vi "Main.vi"() -> ()   [LabVIEW 2017, in "Application.lvlib"]
doc: "This VI is the main application VI in the Delacor QMH project template. This application VI is implemented as a simple state machine, which communicates with two different Delacor QMH modules.\n_____\nBased on Delacor QMH Project Template 3.1.0.34."
uses:
  Application.lvlib
  Application Data--cluster.ctl
  State--enum.ctl
  My Cloneable Module/My Cloneable Module.lvlib
  My Singleton Module/My Singleton Module.lvlib
panel:
  out "version":string
  in  "Hide My Singleton Module":bool
  in  "Show My Singleton Module":bool
  in  "Hide My Cloneable Module":bool
  in  "Show My Cloneable Module":bool
  in  "Stop My Cloneable Module":bool
  in  "Stop My Singleton Module":bool
  in  "Start My Singleton Module":bool
  out "Active Cloneable Modules":string[](array[string])
  in  "Start New Instance My Cloneable Module":bool
  in  "Select Cloneable Module Instance":i32(ring)=-1 items=["All"=-1]
  in  "My Singleton Module: Do Something Else":dbl caption="Do Something Else"
  in  "My Singleton Module: Do Something":bool
  out "My Singleton Running?":bool
  out "Status":string
  in  "My Cloneable Module: Do Something Else":dbl caption="Do Something Else to Selected Module"
  in  "My Cloneable Module: Do Something":bool caption="Do Something to Selected Module"
  # "This top-level application allows you to launch and control a singleton module, and multiple instances of a cloneable module."
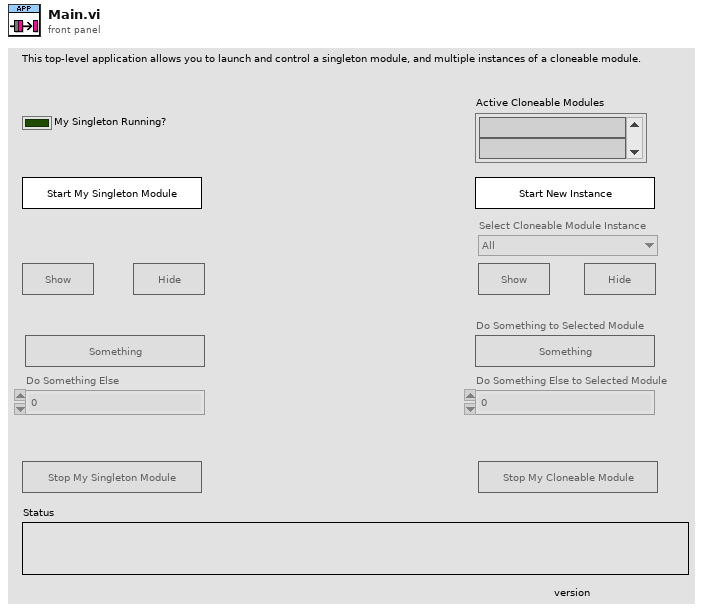
[diagram p1: front panel]
types:
  T1 = typedef "Application.lvlib/State--enum.ctl" = enum16{"Initialize", "Initialize Panel", "UI Interlocks", "Update Status", "Wait for Event", "Exit"}
  T2 = typedef "Application.lvlib/Application Data--cluster.ctl" = cluster{"Status":string, "Singleton Controls":refnum<vi>[], "Cloneable Controls":refnum<vi>[], "Module Ring Value":i32}
  T3 = typedef "My Cloneable Module.lvlib/Broadcast Events--cluster.ctl" = cluster{"Module Did Init":refnum<user-event>, "Status Updated":refnum<user-event>, "Error Reported":refnum<user-event>, "Did Something":refnum<user-event>, "Module Did Stop":refnum<user-event>, "Update Module Execution Status":refnum<user-event>}
  T4 = typedef "My Singleton Module.lvlib/Broadcast Events--cluster.ctl" = cluster{"Module Did Init":refnum<user-event>, "Status Updated":refnum<user-event>, "Error Reported":refnum<user-event>, "Did Something":refnum<user-event>, "Module Did Stop":refnum<user-event>, "Update Module Execution Status":refnum<user-event>}
  T5 = enum8{"Enabled", "Disabled", "Disabled and Grayed Out"}
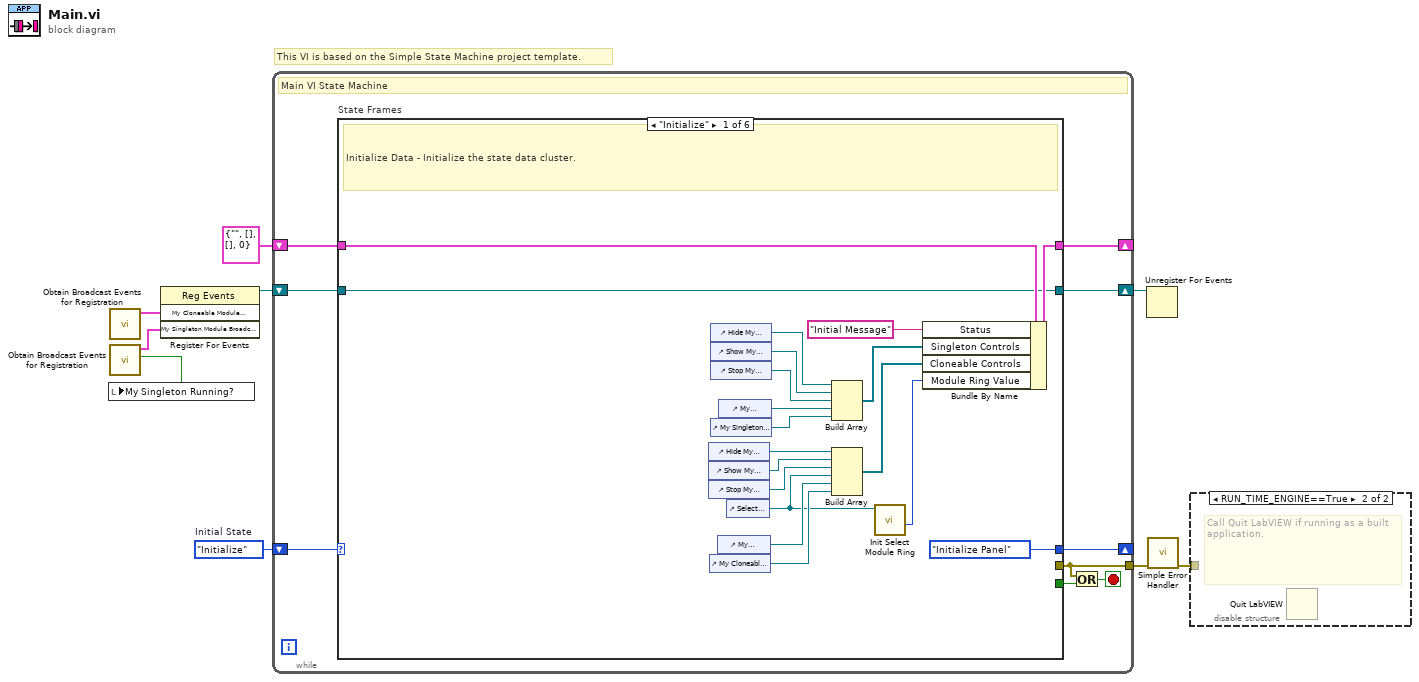
[diagram p0: block diagram]
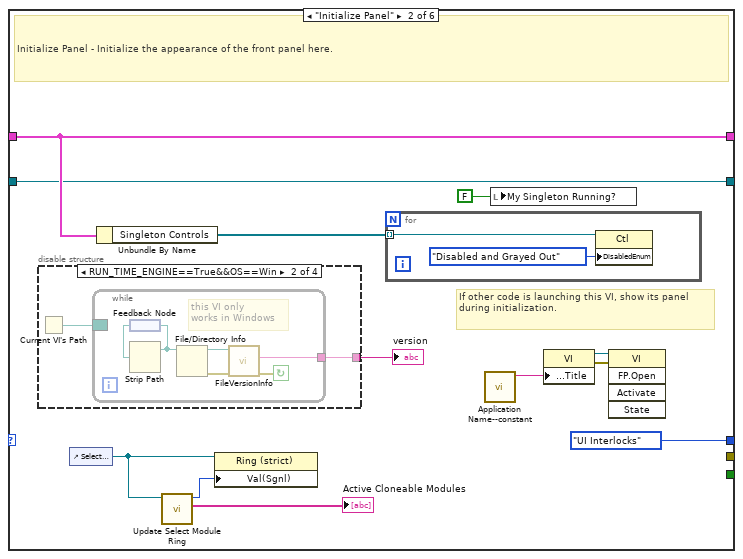
[diagram p2: hidden frame]
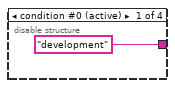
[diagram p3: hidden frame]
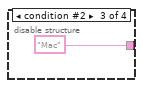
[diagram p4: hidden frame]
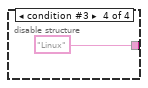
[diagram p5: hidden frame]
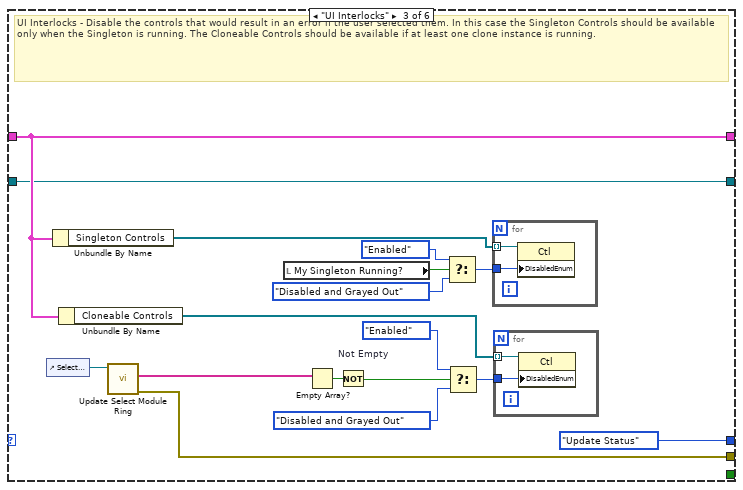
[diagram p6: hidden frame]
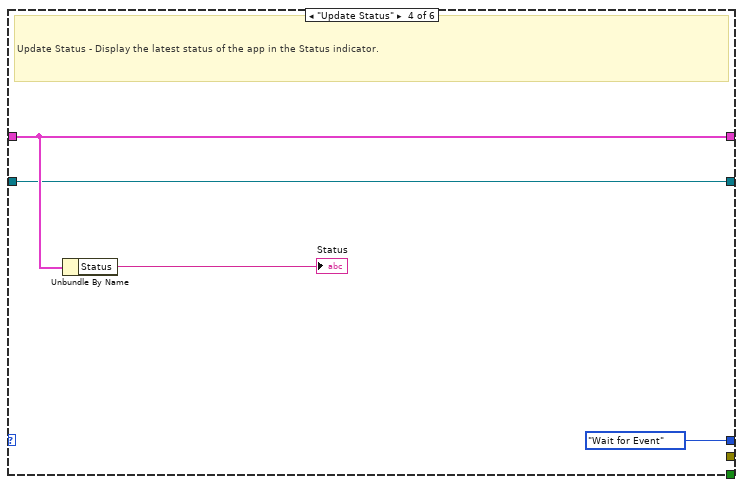
[diagram p7: hidden frame]
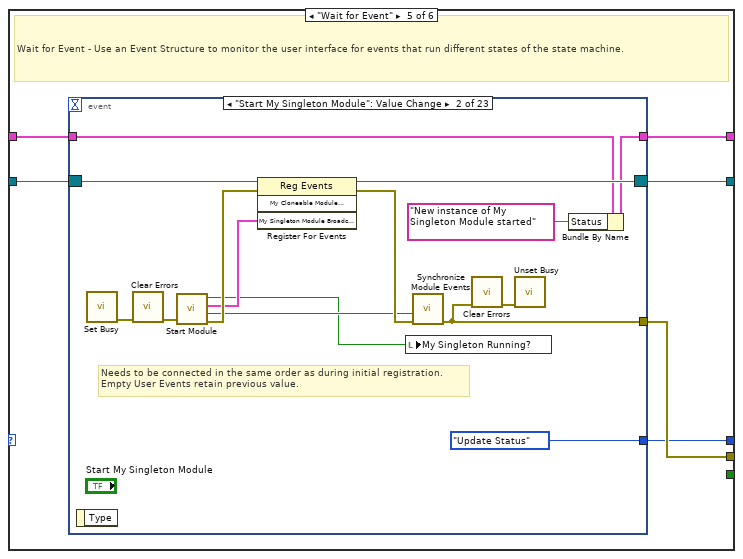
[diagram p8: hidden frame]
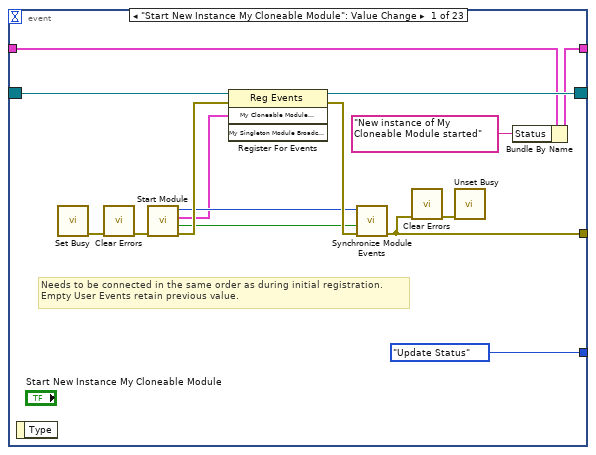
[diagram p9: hidden frame]
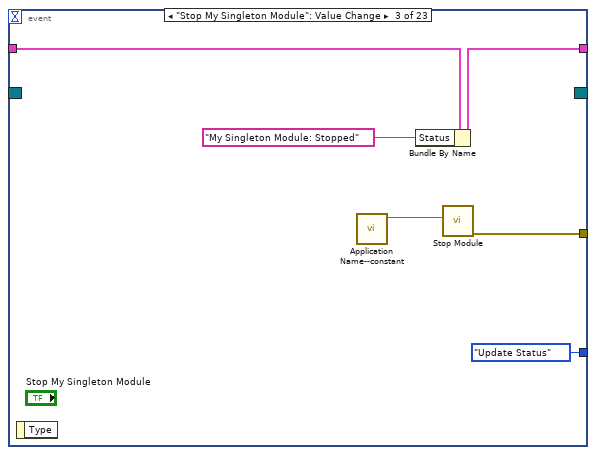
[diagram p10: hidden frame]
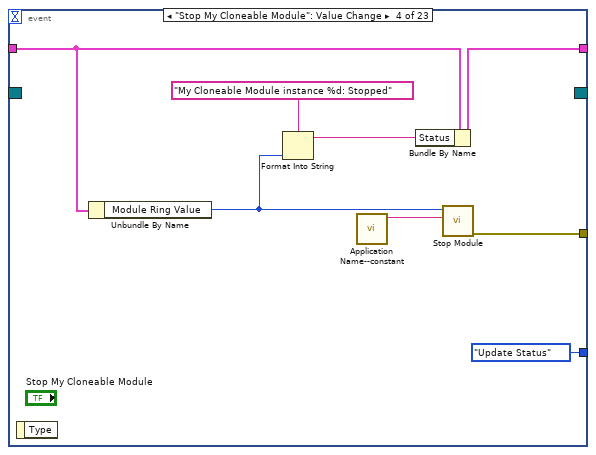
[diagram p11: hidden frame]
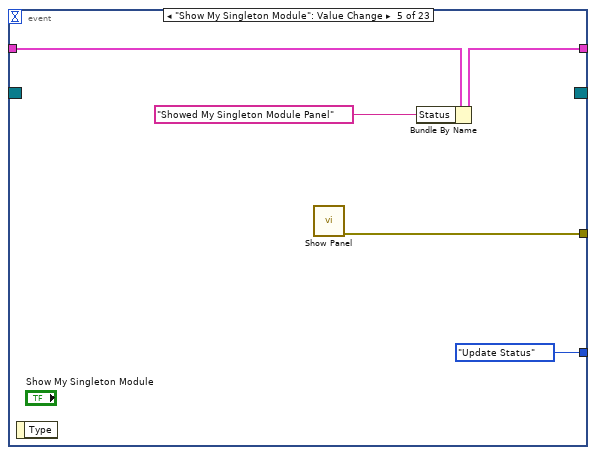
[diagram p12: hidden frame]
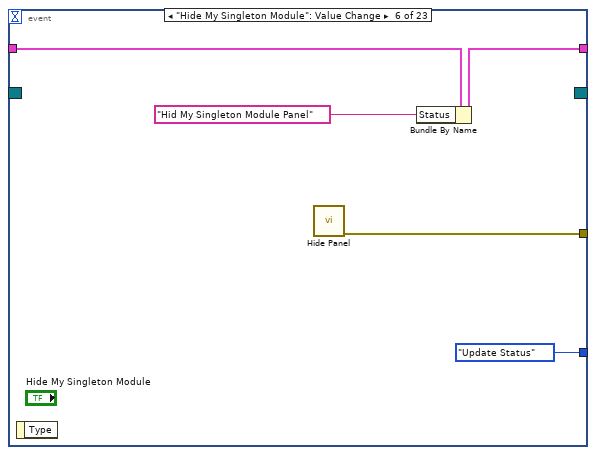
[diagram p13: hidden frame]
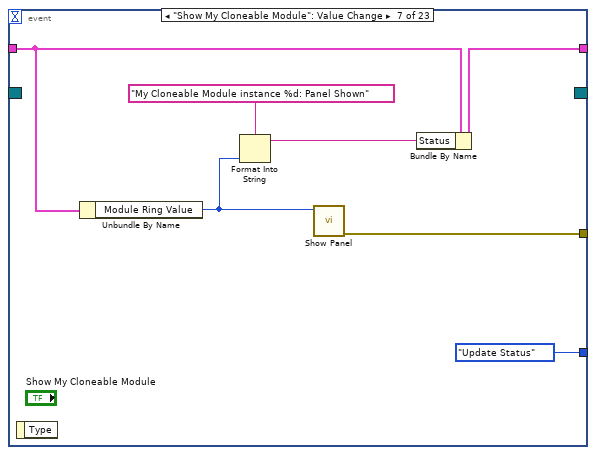
[diagram p14: hidden frame]
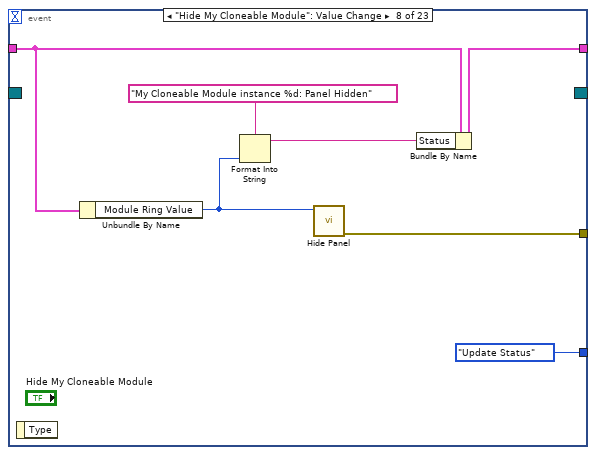
[diagram p15: hidden frame]
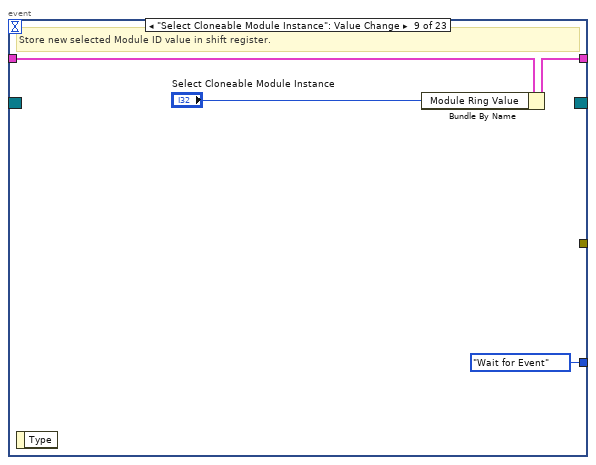
[diagram p16: hidden frame]
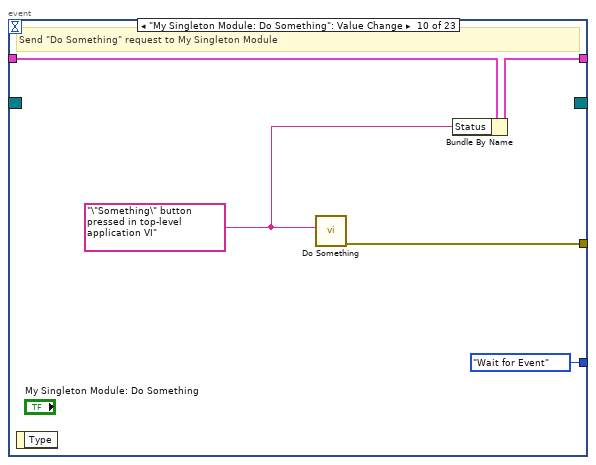
[diagram p17: hidden frame]
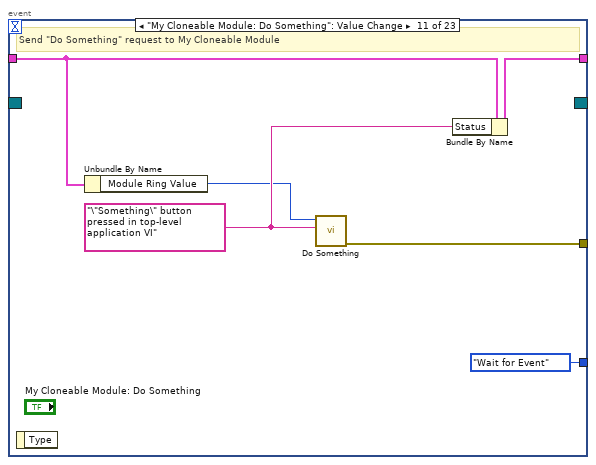
[diagram p18: hidden frame]
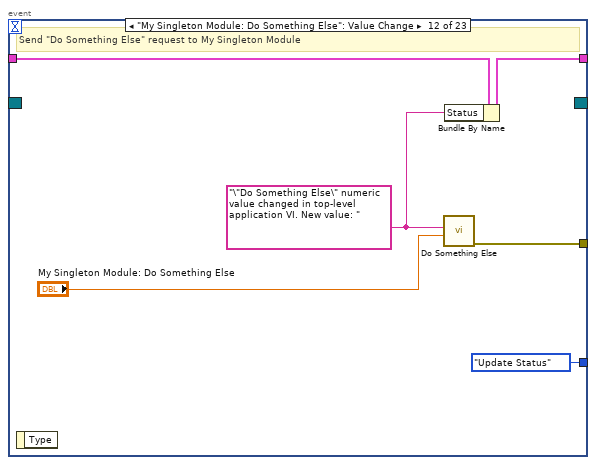
[diagram p19: hidden frame]
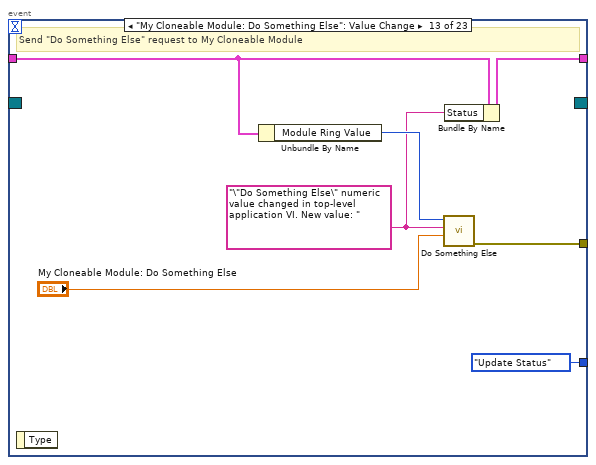
[diagram p20: hidden frame]
diagram:
  w4 = State--enum."Initialize"  # Initial State
  # "This VI is based on the Simple State Machine project template."
  n1 = call "Obtain Broadcast Events for Registration.vi"() -> ("My Cloneable Module Broadcast Events"=w8:T3)  [unwired: 10 in, 1 out]
  n2 = call "Obtain Broadcast Events for Registration.vi"() -> ("Already running?"=w1:bool, "My Singleton Module Broadcast Events"=w7:T4)  [unwired: 9 in, 1 out]
  n3 = local write "My Singleton Running?"(w1) -> ()
  n4 = register-events(w8, w7) -> (reference out=w3:refnum<event-registration>)  [unwired: 2 in, 1 out]
  n5 = while {
    shift-right: [w17] -> _
    shift-left: T2 {"Status"="", "Singleton Controls"=[], "Cloneable Controls"=[], "Module Ring Value"=0} ("Data Cluster") -> [w18]
    tunnel: [w13] -> w6
    shift-right: [w12] -> _
    shift-left: w4 -> [w15]
    shift-right: [w10] -> w2
    shift-left: w3 -> [w11]
    stop <- w14 stop-if-true
    # "Main VI State Machine"
    n6 = case "State Frames" shown="\"Initialize\"" w15 {
      tunnel: [_ _ w63 _ w89 w261] -> w13
      tunnel: w18 -> [w37 w47 w68 w87 w91 w263]
      tunnel: [w36 w47 w68 w87 w90 w263] -> w17
      tunnel: [_ _ _ _ _ w262] -> w16
      tunnel: [State--enum."Initialize Panel" ("State") State--enum."UI Interlocks" ("State") State--enum."Update Status" ("State") State--enum."Wait for Event" ("State") w88 State--enum."Exit" ("State")] -> w12
      tunnel: w11 -> [w19 w44 w64 w84 w93 w257]
      tunnel: [w19 w44 w64 w84 w92 w257] -> w10
      frame "Initialize" {
        # "Initialize Data - Initialize the state data cluster."
        n7 = control-ref of="Hide My Cloneable Module"() -> (w28:refnum<vi>)
        n8 = control-ref of="Show My Cloneable Module"() -> (w27:refnum<vi>)
        n9 = control-ref of="Stop My Cloneable Module"() -> (w26:refnum<vi>)
        n10 = control-ref of="My Cloneable Module: Do Something"() -> (w23:refnum<vi>)
        n11 = control-ref of="Hide My Singleton Module"() -> (w34:refnum<vi>)
        n12 = control-ref of="Show My Singleton Module"() -> (w33:refnum<vi>)
        n13 = control-ref of="Stop My Singleton Module"() -> (w32:refnum<vi>)
        n14 = control-ref of="My Singleton Module: Do Something"() -> (w30:refnum<vi>)
        n15 = control-ref of="My Cloneable Module: Do Something Else"() -> (w24:refnum<vi>)
        n16 = control-ref of="My Singleton Module: Do Something Else"() -> (w31:refnum<vi>)
        n17 = control-ref of="Select Cloneable Module Instance"() -> (w21:refnum<vi>)
        n18 = Build Array(w34, w33, w32, w31, w30) -> (w29:refnum<vi>[])
        n19 = Build Array(w28, w27, w26, w21, w24, w23) -> (w25:refnum<vi>[])
        n20 = call "Init Select Module Ring.vi"("Select Module Ring Ref"=w21) -> ("Module Ring Value"=w20:i32)  [unwired: 8 in, 2 out]
        n21 = Bundle By Name(cluster=w37, "Status"="Initial Message" ("Initial Message"), "Singleton Controls"=w29, "Cloneable Controls"=w25, "Module Ring Value"=w20) -> (w36:T2)
      }
      frame "Initialize Panel" {
        # "If other code is launching this VI, show its panel during initialization."
        # "Initialize Panel - Initialize the appearance of the front panel here."
        n22 = disable-structure "Conditional Disable Structure" shown="RUN_TIME_ENGINE==True&&OS==Win" {
          disable-tunnel: ["development" w51 "Mac" "Linux"] -> w41
          frame condition #0 (active) {
          }
          frame condition #1 {
            n23 = Current VI's Path() -> (path=w52:path)
            n24 = while {
              border: w52 -> [_]
              tunnel: [w53] -> w51
              stop <- w54 continue-if-true
              # "this VI only \nworks in Windows"
              n25 = feedback #1() -> (w58:path)
              n26 = Strip Path(path=w58) -> (stripped path=w57:path)  [unwired: 1 out]
              n27 = feedback-in #1(w57) -> ()
              n28 = File/Directory Info(path=w57) -> (path out=w55:path, error out=w56:errorcluster)  [unwired: 1 in, 5 out]
              n29 = call <vilib>:"FileVersionInfo.vi"("error in (no error)"=w56, "Application Path in"=w55) -> ("error out"=w54:errorcluster, "File Version Info"=w53:string)  [unwired: 6 in, 2 out]
            }
          }
          frame condition #2 {
          }
          frame condition #3 {
          }
        }
        "version" <- w41
        n30 = control-ref of="Select Cloneable Module Instance"() -> (w43:refnum<vi>)
        n31 = Unbundle By Name(w47) -> ("Singleton Controls"=w46:refnum<vi>[])
        n32 = call "Update Select Module Ring.vi"("Select Module Ring Ref"=w43) -> ("Active Modules (Array)"=→"Active Cloneable Modules":string[], "New Module Ring Value"=w42:i32)  [unwired: 8 in, 1 out]
        n33 = property on="Property Node" class="Ring (strict)"(reference=w43, "Val(Sgnl)"=w42) -> ()  [unwired: 1 in, 2 out]
        n34 = for {
          tunnel: w46 -> [w62] mode=indexing
          n35 = property on="Property Node" class="Ctl"(reference=w62, "DisabledEnum"=T5."Disabled and Grayed Out" ("Disabled")) -> ()  [unwired: 1 in, 2 out]
        }
        n36 = call "Application Name--constant.vi"() -> ("Application Name"=w40:string)  [unwired: 11 in]
        n37 = local write "My Singleton Running?"(FALSE ("My Singleton Module Init?")) -> ()
        n38 = property on="Property Node" class="VI"("Front Panel.Title"=w40) -> (reference out=w39:refnum<vi>, error out=w38:errorcluster)  [unwired: 2 in]
        n39 = invoke class="VI" method="FP.Open"(reference=w39, error in=w38) -> ()  [unwired: 3 in, 5 out]
      }
      frame "UI Interlocks" {
        # "UI Interlocks - Disable the controls that would result in an error if the user selected them. In this case the Singleton Controls should be available only when the Singleton is running. The Cloneable Controls should be available if at least one clone instance is running."
        n40 = control-ref of="Select Cloneable Module Instance"() -> (w79:refnum<vi>)
        n41 = Unbundle By Name(w68) -> ("Singleton Controls"=w73:refnum<vi>[])
        n42 = Unbundle By Name(w68) -> ("Cloneable Controls"=w67:refnum<vi>[])
        n43 = call "Update Select Module Ring.vi"("Select Module Ring Ref"=w79) -> ("error out"=w63:errorcluster, "Active Modules (Array)"=w78:string[])  [unwired: 8 in, 1 out]
        n44 = local read "My Singleton Running?"() -> (w72:bool)
        n45 = Empty Array?(array=w78) -> (empty?=w77:bool)
        n46 = Not "Not Empty"(x=w77) -> (.not. x?=w66:bool)
        n47 = Select(t=T5."Enabled" ("Disabled"), s=w72, f=T5."Disabled and Grayed Out" ("Disabled")) -> (s? t:f=w74:T5)
        n48 = Select(t=T5."Enabled" ("Disabled"), s=w66, f=T5."Disabled and Grayed Out" ("Disabled")) -> (s? t:f=w71:T5)
        n49 = for {
          tunnel: w73 -> [w83] mode=indexing
          tunnel: w74 -> [w82]
          n50 = property on="Property Node" class="Ctl"(reference=w83, "DisabledEnum"=w82) -> ()  [unwired: 1 in, 2 out]
        }
        n51 = for {
          tunnel: w67 -> [w81] mode=indexing
          tunnel: w71 -> [w80]
          n52 = property on="Property Node" class="Ctl"(reference=w81, "DisabledEnum"=w80) -> ()  [unwired: 1 in, 2 out]
        }
      }
      frame "Update Status" {
        # "Update Status - Display the latest status of the app in the Status indicator."
        n53 = Unbundle By Name(w87) -> ("Status"=→"Status":string)
      }
      frame "Wait for Event" {
        # "Wait for Event - Use an Event Structure to monitor the user interface for events that run different states of the state machine."
        n54 = event shown="[1] \"Start My Singleton Module\": Value Change" {
          selector: w93 -> [w101 w117 _ _ _ _ _ _ _ _ _ _ _ _ _ _ _ _ _ _ _ _ _]
          dyn-events: [w100 w116 _ _ _ _ _ _ _ _ _ _ _ _ _ _ _ _ _ _ _ _ _] -> w92
          timeout: _ -> [_ _ _ _ _ _ _ _ _ _ _ _ _ _ _ _ _ _ _ _ _ _ _]
          tunnel: [w108 w123 w127 w135 w142 w147 w154 w161 _ w170 w176 w182 w189 w193 w198 w204 _ _ _ _ w241 _ _] -> w89
          tunnel: [w96 w113 w125 w134 w140 w145 w153 w160 w163 w168 w175 w180 w188 w192 w200 w206 w207 w212 w223 w233 w236 w247 w252] -> w90
          tunnel: w91 -> [w97 w114 w126 w133 w141 w146 w151 w158 w164 w169 w172 w181 w186 w192 w200 w206 w208 w213 w224 w234 w239 w248 w252]
          tunnel: [State--enum."Update Status" ("State") State--enum."Update Status" ("State") State--enum."Update Status" ("State") State--enum."Update Status" ("State") State--enum."Update Status" ("State") State--enum."Update Status" ("State") State--enum."Update Status" ("State") State--enum."Update Status" ("State") State--enum."Wait for Event" ("State") State--enum."Wait for Event" ("State") State--enum."Wait for Event" ("State") State--enum."Update Status" ("State") State--enum."Update Status" ("State") State--enum."UI Interlocks" ("State") State--enum."UI Interlocks" ("State") State--enum."UI Interlocks" ("State") State--enum."Update Status" ("State") State--enum."Update Status" ("State") State--enum."Update Status" ("State") State--enum."Update Status" ("State") State--enum."UI Interlocks" ("State") State--enum."UI Interlocks" ("State") State--enum."Exit" ("State")] -> w88
          event "Start New Instance My Cloneable Module": Value Change {
            # "Needs to be connected in the same order as during initial registration.\nEmpty User Events retain previous value."
            n55 = event-data() -> ()  [unwired: 1 in, 1 out]
            n56 = call <vilib>:"Set Busy.vi"() -> ("error out"=w102:errorcluster)  [unwired: 10 in, 1 out]
            n57 = call <vilib>:"Clear Errors.vi"("error in (no error)"=w102) -> ("error out"=w103:errorcluster)  [unwired: 5 in, 1 out]
            n58 = call "Start Module.vi"("error in (no error)"=w103) -> ("error out"=w107:errorcluster, "Wait for Event Sync?"=w105:bool, "My Cloneable Module Broadcast Events"=w99:T3, "Module ID"=w104:i32)  [unwired: 7 in]
            n59 = register-events(reference=w101, error in=w107, w99) -> (reference out=w100:refnum<event-registration>, error out=w106:errorcluster)  [unwired: 1 in]
            n60 = call "Synchronize Module Events.vi"("error in (no error)"=w106, "Wait for Event Sync?"=w105, "Module ID"=w104) -> ("error out"=w108:errorcluster)  [unwired: 7 in, 1 out]
            n61 = call <vilib>:"Clear Errors.vi"("error in (no error)"=w108) -> ("error out"=w94:errorcluster)  [unwired: 5 in, 1 out]
            n62 = call <vilib>:"Unset Busy.vi"("error in (no error)"=w94) -> ()  [unwired: 10 in, 1 out]
            n63 = Bundle By Name(cluster=w97, "Status"="New instance of My Cloneable Module started") -> (w96:T2)
          }
          event "Start My Singleton Module": Value Change {
            # "Needs to be connected in the same order as during initial registration.\nEmpty User Events retain previous value."
            n64 = event-data() -> ()  [unwired: 1 in, 1 out]
            n65 = call <vilib>:"Set Busy.vi"() -> ("error out"=w118:errorcluster)  [unwired: 10 in, 1 out]
            n66 = call <vilib>:"Clear Errors.vi"("error in (no error)"=w118) -> ("error out"=w119:errorcluster)  [unwired: 5 in, 1 out]
            n67 = call "Start Module.vi"("error in (no error)"=w119) -> ("error out"=w122:errorcluster, "Wait for Event Sync?"=w120:bool, "My Singleton Module Broadcast Events"=w111:T4, "Module Was Already Running?"=w109:bool)  [unwired: 7 in]
            n68 = register-events(reference=w117, error in=w122, w111) -> (reference out=w116:refnum<event-registration>, error out=w121:errorcluster)  [unwired: 1 in]
            n69 = local write "My Singleton Running?"(w109) -> ()
            n70 = call "Synchronize Module Events.vi"("error in (no error)"=w121, "Wait for Event Sync?"=w120) -> ("error out"=w123:errorcluster)  [unwired: 9 in]
            n71 = call <vilib>:"Clear Errors.vi"("error in (no error)"=w123) -> ("error out"=w110:errorcluster)  [unwired: 5 in, 1 out]
            n72 = call <vilib>:"Unset Busy.vi"("error in (no error)"=w110) -> ()  [unwired: 10 in, 1 out]
            n73 = Bundle By Name(cluster=w114, "Status"="New instance of My Singleton Module started") -> (w113:T2)
          }
          event "Stop My Singleton Module": Value Change {
            n74 = event-data() -> ()  [unwired: 1 in, 1 out]
            n75 = call "Application Name--constant.vi"() -> ("Application Name"=w128:string)  [unwired: 11 in]
            n76 = Bundle By Name(cluster=w126, "Status"="My Singleton Module: Stopped" ("Message")) -> (w125:T2)
            n77 = call "Stop Module.vi"("Origin"=w128) -> ("error out"=w127:errorcluster)  [unwired: 10 in]
          }
          event "Stop My Cloneable Module": Value Change {
            n78 = event-data() -> ()  [unwired: 1 in, 1 out]
            n79 = Unbundle By Name(w133) -> ("Module Ring Value"=w130:i32)
            n80 = Format Into String(format string="My Cloneable Module instance %d: Stopped" ("Message"), w130) -> (resulting string=w131:string)  [unwired: 2 in, 1 out]
            n81 = call "Application Name--constant.vi"() -> ("Application Name"=w136:string)  [unwired: 11 in]
            n82 = Bundle By Name(cluster=w133, "Status"=w131) -> (w134:T2)
            n83 = call "Stop Module.vi"("Origin"=w136, "Module ID"=w130) -> ("error out"=w135:errorcluster)  [unwired: 9 in]
          }
          event "Show My Singleton Module": Value Change {
            n84 = event-data() -> ()  [unwired: 1 in, 1 out]
            n85 = call "Show Panel.vi"() -> ("error out"=w142:errorcluster)  [unwired: 11 in]
            n86 = Bundle By Name(cluster=w141, "Status"="Showed My Singleton Module Panel" ("Message")) -> (w140:T2)
          }
          event "Hide My Singleton Module": Value Change {
            n87 = event-data() -> ()  [unwired: 1 in, 1 out]
            n88 = call "Hide Panel.vi"() -> ("error out"=w147:errorcluster)  [unwired: 11 in]
            n89 = Bundle By Name(cluster=w146, "Status"="Hid My Singleton Module Panel" ("Message")) -> (w145:T2)
          }
          event "Show My Cloneable Module": Value Change {
            n90 = event-data() -> ()  [unwired: 1 in, 1 out]
            n91 = Unbundle By Name(w151) -> ("Module Ring Value"=w149:i32)
            n92 = Format Into String(format string="My Cloneable Module instance %d: Panel Shown" ("Message"), w149) -> (resulting string=w148:string)  [unwired: 2 in, 1 out]
            n93 = call "Show Panel.vi"("Module ID"=w149) -> ("error out"=w154:errorcluster)  [unwired: 10 in]
            n94 = Bundle By Name(cluster=w151, "Status"=w148) -> (w153:T2)
          }
          event "Hide My Cloneable Module": Value Change {
            n95 = event-data() -> ()  [unwired: 1 in, 1 out]
            n96 = Unbundle By Name(w158) -> ("Module Ring Value"=w156:i32)
            n97 = Format Into String(format string="My Cloneable Module instance %d: Panel Hidden" ("Message"), w156) -> (resulting string=w155:string)  [unwired: 2 in, 1 out]
            n98 = call "Hide Panel.vi"("Module ID"=w156) -> ("error out"=w161:errorcluster)  [unwired: 10 in]
            n99 = Bundle By Name(cluster=w158, "Status"=w155) -> (w160:T2)
          }
          event "Select Cloneable Module Instance": Value Change {
            # "Store new selected Module ID value in shift register."
            n100 = event-data() -> ()  [unwired: 1 in, 1 out]
            n101 = Bundle By Name(cluster=w164, "Module Ring Value"="Select Cloneable Module Instance") -> (w163:T2)
          }
          event "My Singleton Module: Do Something": Value Change {
            w167 = "\"Something\" button pressed in top-level application VI" ("\"Do Something Else\" button pressed")
            # "Send \"Do Something\" request to My Singleton Module"
            n102 = event-data() -> ()  [unwired: 1 in, 1 out]
            n103 = call "Do Something.vi"("Do Something Message"=w167) -> ("error out"=w170:errorcluster)  [unwired: 10 in]
            n104 = Bundle By Name(cluster=w169, "Status"=w167) -> (w168:T2)
          }
          event "My Cloneable Module: Do Something": Value Change {
            w174 = "\"Something\" button pressed in top-level application VI" ("\"Do Something Else\" button pressed")
            # "Send \"Do Something\" request to My Cloneable Module"
            n105 = event-data() -> ()  [unwired: 1 in, 1 out]
            n106 = Unbundle By Name(w172) -> ("Module Ring Value"=w171:i32)
            n107 = call "Do Something.vi"("Do Something Message"=w174, "Module ID"=w171) -> ("error out"=w176:errorcluster)  [unwired: 9 in]
            n108 = Bundle By Name(cluster=w172, "Status"=w174) -> (w175:T2)
          }
          event "My Singleton Module: Do Something Else": Value Change {
            w177 = "\"Do Something Else\" numeric value changed in top-level application VI. New value: " ("\"Do Something Else\" button pressed")
            # "Send \"Do Something Else\" request to My Singleton Module"
            n109 = event-data() -> ()  [unwired: 1 in, 1 out]
            n110 = call "Do Something Else.vi"("X"="My Singleton Module: Do Something Else", "Do Something Else Message"=w177) -> ("error out"=w182:errorcluster)  [unwired: 9 in]
            n111 = Bundle By Name(cluster=w181, "Status"=w177) -> (w180:T2)
          }
          event "My Cloneable Module: Do Something Else": Value Change {
            w183 = "\"Do Something Else\" numeric value changed in top-level application VI. New value: " ("\"Do Something Else\" button pressed")
            # "Send \"Do Something Else\" request to My Cloneable Module"
            n112 = event-data() -> ()  [unwired: 1 in, 1 out]
            n113 = Unbundle By Name(w186) -> ("Module Ring Value"=w185:i32)
            n114 = call "Do Something Else.vi"("X"="My Cloneable Module: Do Something Else", "Do Something else Message"=w183, "Module ID"=w185) -> ("error out"=w189:errorcluster)  [unwired: 8 in]
            n115 = Bundle By Name(cluster=w186, "Status"=w183) -> (w188:T2)
          }
          event User Event {
            # "A new instance of My Cloneable Module has broadcast that is has been initialized"
            n116 = event-data() -> ("Info"=w197:string, "Module ID"=w191:i32)  [unwired: 1 in]
            n117 = local write "Status"(w197) -> ()
            n118 = control-ref of="Select Cloneable Module Instance"() -> (w196:refnum<vi>)
            n119 = call "Update Select Module Ring.vi"("Select Module Ring Ref"=w196) -> ("error out"=w190:errorcluster, "Active Modules (Array)"=w195:string[])  [unwired: 8 in, 1 out]
            n120 = local write "Active Cloneable Modules"(w195) -> ()
            n121 = call "Show Panel.vi"("error in (no error)"=w190, "Module ID"=w191) -> ("error out"=w193:errorcluster)  [unwired: 9 in]
          }
          event User Event {
            # "My Singleton Module has broadcast that it has been initialized"
            n122 = event-data() -> ("Init?"=→"My Singleton Running?":bool, "Info"=w202:string)  [unwired: 1 in]
            n123 = local write "Status"(w202) -> ()
            n124 = call "Show Panel.vi"() -> ("error out"=w198:errorcluster)  [unwired: 11 in]
          }
          event User Event {
            # "My Singleton Module has broadcast its execution status"
            n125 = event-data() -> ("Running?"=w203:bool)  [unwired: 1 in]
            n126 = local write "My Singleton Running?"(w203) -> ()
            n127 = call "Show Panel.vi"() -> ("error out"=w204:errorcluster)  [unwired: 11 in]
          }
          event User Event {
            # "An instance of My Cloneable Module has broadcast its status"
            n128 = event-data() -> ("Status"=w210:string)  [unwired: 1 in]
            n129 = Bundle By Name(cluster=w208, "Status"=w210) -> (w207:T2)
          }
          event User Event {
            # "My Singleton Module has broadcast its status"
            n130 = event-data() -> ("Status"=w214:string)  [unwired: 1 in]
            n131 = Bundle By Name(cluster=w213, "Status"=w214) -> (w212:T2)
          }
          event User Event {
            # "My Cloneable Module had an error"
            n132 = event-data() -> ("Module Name"=w216:string, "Additional Information"=w219:string, "Error"=w220:errorcluster)  [unwired: 1 in]
            n133 = Unbundle By Name(w220) -> ("code"=w215:i32, "source"=w218:string)
            n134 = Format Into String(format string="Error code %d  Module: %s Additional Information: %s\nSource: %s", w215, w216, w219, w218) -> (resulting string=w217:string)  [unwired: 2 in, 1 out]
            n135 = Bundle By Name(cluster=w224, "Status"=w217) -> (w223:T2)
          }
          event User Event {
            # "My Singleton Module had an error"
            n136 = event-data() -> ("Module Name"=w226:string, "Additional Information"=w231:string, "Error"=w230:errorcluster)  [unwired: 1 in]
            n137 = Unbundle By Name(w230) -> ("code"=w225:i32, "source"=w229:string)
            n138 = Format Into String(format string="Error code %d Module: %s  Additional Information: %s\nSource: %s", w225, w226, w231, w229) -> (resulting string=w227:string)  [unwired: 2 in, 1 out]
            n139 = Bundle By Name(cluster=w234, "Status"=w227) -> (w233:T2)
          }
          event User Event {
            n140 = event-data() -> ("Origin"=w238:string)  [unwired: 1 in]
            n141 = Bundle By Name(cluster=w239, "Status"=w238) -> (w237:T2)
            n142 = control-ref of="Select Cloneable Module Instance"() -> (w243:refnum<vi>)
            n143 = call "Update Select Module Ring.vi"("Select Module Ring Ref"=w243) -> ("error out"=w241:errorcluster, "Active Modules (Array)"=w242:string[], "New Module Ring Value"=w235:i32)  [unwired: 8 in]
            n144 = Bundle By Name(cluster=w237, "Module Ring Value"=w235) -> (w236:T2)
            n145 = local write "Active Cloneable Modules"(w242) -> ()
          }
          event User Event {
            n146 = event-data() -> ("Origin"=w245:string)  [unwired: 1 in]
            n147 = local write "My Singleton Running?"(FALSE ("My Singleton Module Init?")) -> ()
            n148 = Concatenate Strings(w245, " Did Stop.") -> (w244:string)
            n149 = Bundle By Name(cluster=w248, "Status"=w244) -> (w247:T2)
          }
          event Panel Close? {
            # "Go to the 'Exit' state if the user tries to close the panel."
            n150 = event-data() -> ()  [unwired: 1 in, 1 out]
            n151 = event-data ("Event Filter Node")("Discard?"=TRUE) -> ()  [unwired: 1 in, 1 out]
          }
        }
      }
      frame "Exit" {
        w254 = TRUE  # Wait for Module to stop?
        w262 = TRUE  # Stop the VI
        # "Stop all modules launched"
        # "Exit - Exit the application."
        n152 = call "Application Name--constant.vi"() -> ("Application Name"=w255:string)  [unwired: 11 in]
        n153 = call "Stop Module.vi"("Wait for Module to stop? (F)"=w254, "Origin"=w255, "Module ID"=-1) -> ("error out"=w259:errorcluster)  [unwired: 8 in]
        n154 = call "Stop Module.vi"("Wait for Module to Stop? (F)"=w254, "Origin"=w255) -> ("error out"=w260:errorcluster)  [unwired: 9 in]
        n155 = Merge Errors(w259, w260) -> (w261:errorcluster)
      }
    }
    n156 = Or(x=w13, y=w16) -> (x .or. y?=w14:bool)
  }
  n157 = Unregister For Events(event registration refnum=w2) -> ()  [unwired: 1 in, 1 out]
  n158 = call <vilib>:"Simple Error Handler.vi"("error in (no error)"=w6) -> ("error out"=w5:errorcluster)  [unwired: 4 in, 4 out]
  n159 = disable-structure "Conditional Disable Structure" shown="RUN_TIME_ENGINE==True" {
    disable-tunnel: w5 -> [_ _]
    frame condition #0 (active) {
    }
    frame condition #1 {
      # "Call Quit LabVIEW if running as a built application."
      n160 = Quit LabVIEW() -> ()  [unwired: 1 in]
    }
  }
